vi "Get Data from FIFO (2x) U512 to U256.vi"(4 "Ready for Output":bool, 7 "FIFO In":refnum<k21>="FIFO (U512)") -> (0 "Data Valid":bool, 3 "Output Data":i16[](array[numeric]))   [LabVIEW 2012]
doc: "<b>This VI reads data from a FIFO and transfers data to downstream node in 2 Ticks</b>"
uses:
  <vilib>/rvi/Emulation/niFpgaSctlEmulationGetInTimedLoop.vi
  <vilib>/rvi/DataTransferAndStorage/Container/Common/niFpgaContainerExecOnDevCompGetState.vi
  <vilib>/rvi/DataTransferAndStorage/Container/Common/niFpgaContainerGetUniqueNameForEmu.vi
  <vilib>/rvi/FIFO/Fifo_Resource/nirvififoEmulationSetSize.vi
  <vilib>/rvi/Emulation/niFpgaSctlEmulationFifoFullMgr.vi
  <vilib>/rvi/errors/niFpgaSetErrorForExecOnDevCompSimple.vi
  <vilib>/rvi/eio/common/nirviEmuReportErrorAndStop.vi
  <vilib>/rvi/interface/RandomDataEmulation/nirviRandomDataFPGAFIFO.vi
  <vilib>/rvi/interface/RandomDataEmulation/niFpgaRandomDataHandleErrors.vi
  <vilib>/rvi/DataTransferAndStorage/Container/XNode/niFpgaContainer.xnode
  <vilib>/rvi/FIFO/Fifo_Resource/niFpgaFifoEmulationRefIn.vi
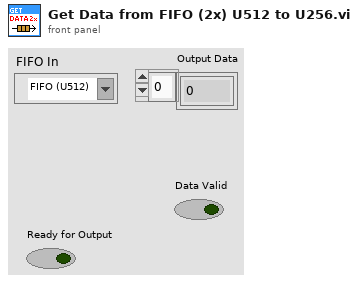
[diagram p1: front panel]
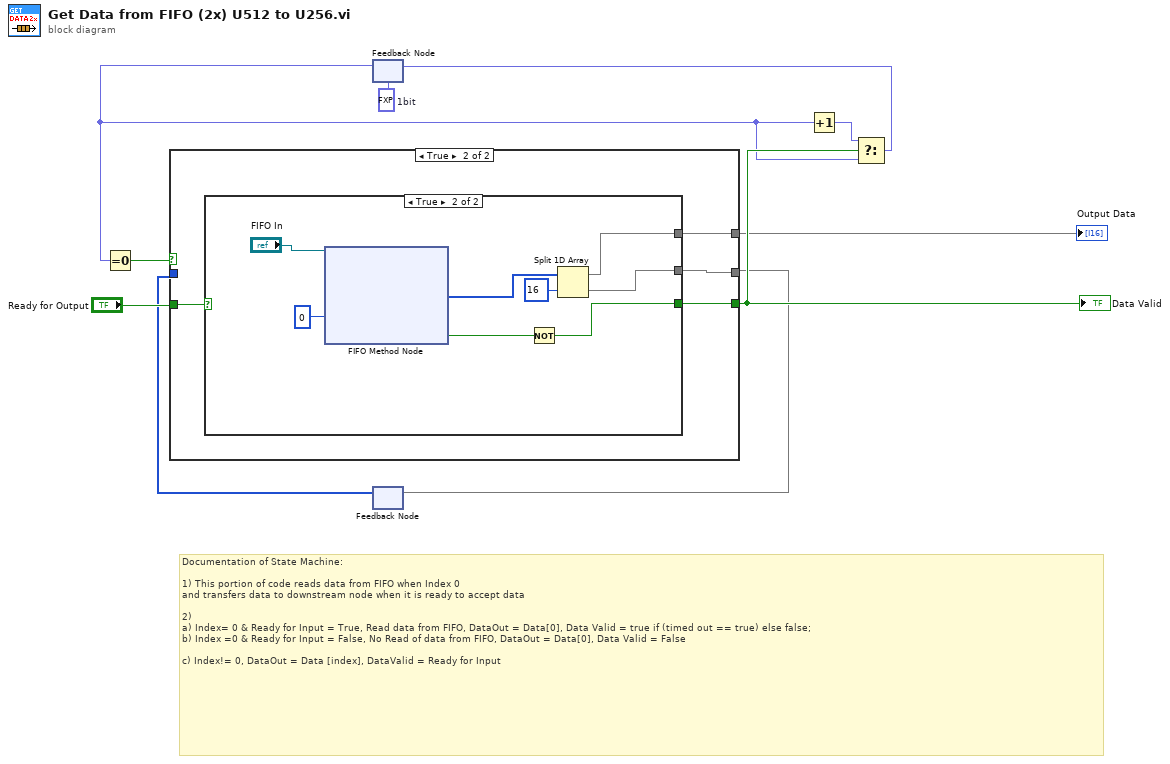
[diagram p0: block diagram]
diagram:
  w4 = fxp<+,1,1> 0.0  # 1bit
  # "Documentation of State Machine:\n\n1) This portion of code reads data from FIFO when Index 0\nand transfers data to downstream node when it is ready to accept data\n\n2) \na) Index= 0 & Ready for Input = True, Read data from FIFO, DataOut = Data[0], Data Valid = true if (timed out == true) else false; \nb) Index =0 & Ready for Input = False, No Read of data from FIFO, DataOut = Data[0], Data Valid = False\n\nc) Index!= 0, DataOut = Data [index], DataValid = Ready for Input"
  n1 = feedback #1(w4) -> (w8:fxp<+,1,1>)
  n2 = Equal To 0?(x=w8) -> (x = 0?=w5:bool)
  n3 = feedback #2() -> (w2:i16[])  [unwired: 1 in]
  n4 = case shown="True" w5 {
    tunnel: [w12 w15] -> w9
    tunnel: [w11 w16] -> w3
    tunnel: w2 -> [w11 _]
    tunnel: "Ready for Output" -> [w12 w14]
    tunnel: [w11 w13] -> w1
    frame False {
    }
    frame True {
      n5 = case shown="True" w14 {
        tunnel: [_ w19] -> w16
        tunnel: [_ w24] -> w15
        tunnel: [_ w17] -> w13
        frame False {
        }
        frame True {
          n6 = xnode ("FIFO Method Node")("Timeout"=0, "FIFO In"="FIFO In") -> ("Element"=w20:i16[], "Timed Out?"=w22:bool)  [unwired: 1 out]
          n7 = Not(x=w22) -> (.not. x?=w24:bool)
          n8 = Split 1D Array(array=w20, index=16) -> (first subarray=w17:i16[], second subarray=w19:i16[])
        }
      }
    }
  }
  "Data Valid" <- w9
  "Output Data" <- w1
  n9 = feedback-in #2(w3) -> ()
  n10 = Increment(x=w8) -> (x+1=w6:fxp<+,1,1>)
  n11 = Select(t=w6, s=w9, f=w8) -> (s? t:f=w7:fxp<+,1,1>)
  n12 = feedback-in #1(w7) -> ()
